vi "arrayTo_Graph_syncCh.vi"(8 "error in (no error)":errorcluster, 9 "Timebase frequency":dbl format="%#_13g", 10 "Timestamp start":dbl format="%#_13g", 11 "Data":variant[](array[variant])) -> (0 "error out":errorcluster, 3 "Data":T1)   [LabVIEW 2020, in "OXYGEN_Datastream.lvlib"]
uses:
  OXYGEN_Datastream.lvlib
  TypeDefs/DataPoint_Variant.ctl
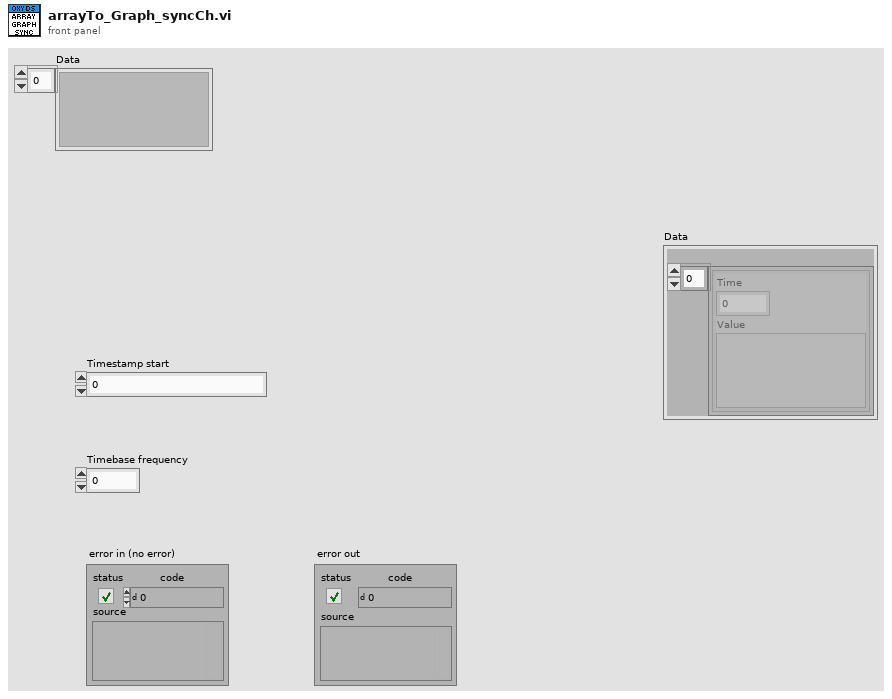
[diagram p1: front panel]
types:
  T1 = typedef "OXYGEN_Datastream.lvlib/DataPoint_Variant.ctl" = cluster{"DataPoints":cluster{"Time":dbl, "Value":variant}[]}
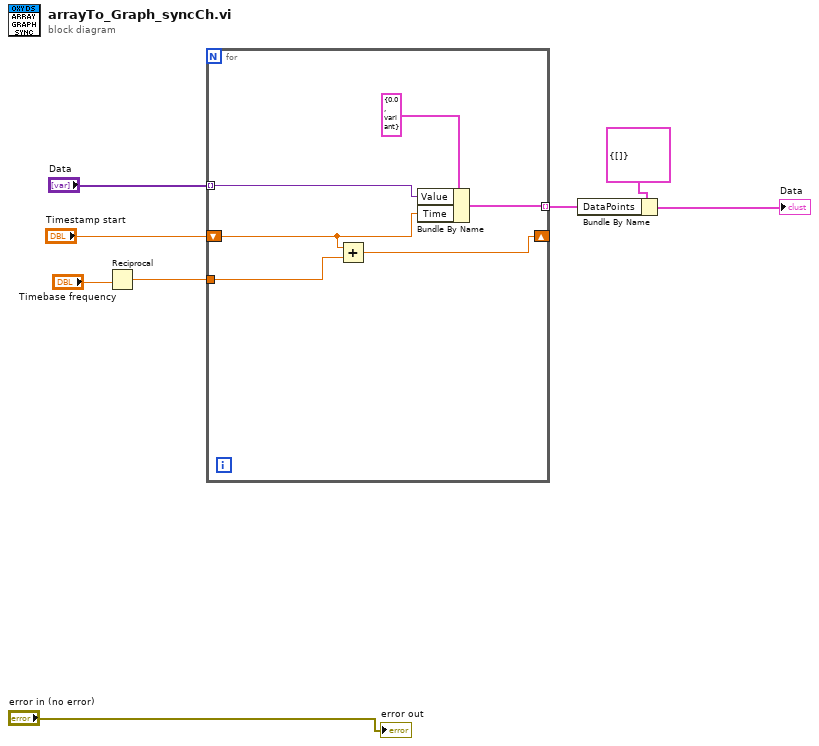
[diagram p0: block diagram]
diagram:
  n1 = Reciprocal(x="Timebase frequency") -> (1/x=w7:dbl)
  n2 = for {
    tunnel: w7 -> [w14]
    shift-right: [w13] -> _
    shift-left: "Timestamp start" -> [w9]
    tunnel: "Data" -> [w10] mode=indexing
    tunnel: [w12] -> w2 mode=indexing
    n3 = Add(x=w9, y=w14) -> (x+y=w13:dbl)
    n4 = Bundle By Name(cluster=cluster{"Time":dbl, "Value":variant} {"Time"=0.0, "Value"=variant}, "Value"=w10, "Time"=w9) -> (w12:cluster{"Time":dbl, "Value":variant})
  }
  n5 = Bundle By Name(cluster=T1 {"DataPoints"=[]} ("Data"), "DataPoints"=w2) -> (→"Data":T1)
  "error out" <- "error in (no error)"
